vi "Main.vi"() -> ()   [LabVIEW 2018] (continued)
                    n1254 = call "SQL_Update.vi"("查询语句"=w6511, "表名"="Online", "error in (no error)"=w6514, "列名对应的值"=w6512, "列名"=string[] ["Last_Station", "Last_Result", "ST602_Date", "ST602_Time", "ST602_Result", "ST602_PanelNumber"], "connection reference"=w6513) -> ("error out"=w6510:errorcluster)  [unwired: 4 in, 1 out]
                    n1255 = Unbundle By Name(w6510) -> ("status"=w6518:bool)
                    n1256 = Equal?(x=w6509, y="") -> (x = y?=w6516:bool)
                    n1257 = Or(x=w6518, y=w6516) -> (x .or. y?=w6515:bool)
                    n1258 = case shown="假" w6515 {
                      tunnel: ["1" ("数据保存请求回复") "2" ("数据保存请求回复")] -> w6508
                      frame False {
                      }
                      frame True {
                      }
                    }
                  }
                  frame True {
                    n1259 = Delete From Array(array=w6539, length=2 ("长度"), index=0 ("索引")) -> (deleted portion=w6527:string[], array with subset deleted=w6536:string[])
                    n1260 = call "SQL_Update.vi"("查询语句"=w6524, "表名"="Online", "error in (no error)"=w6532, "列名对应的值"=w6527, "列名"=string[] ["Last_Station", "Last_Result"], "connection reference"=w6533) -> ("error out"=w6531:errorcluster, "connection reference 2"=w6530:T5)  [unwired: 4 in]
                    n1261 = call "SQL_Update.vi"("查询语句"=w6524, "表名"="Rework", "error in (no error)"=w6531, "列名对应的值"=w6536, "列名"=string[] ["ST602_Date", "ST602_Time", "ST602_Result", "ST602_PanelNumber"], "connection reference"=w6530) -> ("error out"=w6525:errorcluster)  [unwired: 4 in, 1 out]
                    n1262 = Unbundle By Name(w6525) -> ("status"=w6542:bool)
                    n1263 = Equal?(x="", y=w6534) -> (x = y?=w6541:bool)
                    n1264 = Or(x=w6542, y=w6541) -> (x .or. y?=w6540:bool)
                    n1265 = case shown="真" w6540 {
                      tunnel: ["1" ("数据保存请求回复") "2" ("数据保存请求回复")] -> w6526
                      frame False {
                      }
                      frame True {
                      }
                    }
                  }
                }
              }
            }
            "数据保存请求回复602" <- w6455
            n1266 = Delete From Array(array=w6443, length=2 ("长度"), index=0 ("索引")) -> (array with subset deleted=w6450:string[])  [unwired: 1 out]
            n1267 = local write "602数据回复输入"(w6454) -> ()
            n1268 = Insert Into Array(array=w6450, index=2 ("索引"), new element=w6442) -> (w6449:string[])
            n1269 = Insert Into Array(array=string[][] [] ("数组"), index (row)=0 ("索引 (行)"), new element=w6449) -> (w6451:string[][])  [unwired: 1 in]
            n1270 = Transpose 2D Array(2D array=w6451) -> (transposed array=w6441:string[][])
            n1271 = property on="ST602_DATA" class="MCListbox (严格)"("ItemNames"=w6441) -> ()  [unwired: 2 in, 2 out]
            "ST602数据读取（事件）" <- FALSE ("ST602数据读取（事件）")
          }
          event "ST603扫码请求（事件）": Value Change {
            n1272 = event-data() -> ()  [unwired: 1 in, 2 out]
            n1273 = local read "603二维码"() -> (w6548:string)
            n1274 = Concatenate Strings("Where QRCode='" ("查询语句"), w6548, "'" ("字符串")) -> (w6559:string)
            n1275 = call "SQL_Select.vi"("要读取的列名"=string[] ["Last_Station", "Last_Result"], "表名"="Online", "error in (no error)"=w6551, "查询语句"=w6559, "查询条件"=TRUE, "connection reference"=w6552) -> ("error out"=w6550:errorcluster, "数据"=w6558:string[][])  [unwired: 3 in, 1 out]
            n1276 = case shown="无错误" w6550 {
              tunnel: w6558 -> [w6568 _]
              tunnel: ["1" ("右扫码请求回复") "2" ("右扫码请求回复")] -> w6547
              tunnel: [TRUE TRUE] -> w6546
              frame No Error {
                n1277 = Index Array(array=w6568, index (row)=0 ("索引 (行)")) -> (element=w6565:string[])  [unwired: 1 in]
                n1278 = Index Array(array=w6565, index #1=0 ("索引 (行)")) -> (element #1=→"上一站号 (603)":string, element #2=→"上一站结果 (603)":string)  [unwired: 1 in]
              }
              frame Error {
              }
            }
            "扫码请求回复603" <- w6547
            n1279 = local write "603扫码回复输入"(w6546) -> ()
            "ST603扫码请求（事件）" <- FALSE ("ST603扫码请求（事件）")
          }
          event "ST603数据读取（事件）": Value Change {
            w6593 = 0 ("索引 (行)")
            n1280 = event-data() -> ()  [unwired: 1 in, 2 out]
            n1281 = local read "603二维码"() -> (w6572:string)
            n1282 = Concatenate Strings("Where QRCode='" ("查询语句"), w6572, "'" ("字符串")) -> (w6600:string)
            n1283 = call "SQL_Select.vi"("要读取的列名"=string[] ["Rework_Status"], "表名"="Online", "error in (no error)"=w6586, "查询语句"=w6600, "查询条件"=TRUE, "connection reference"=w6587) -> ("error out"=w6595:errorcluster, "数据"=w6599:string[][], "connection reference out"=w6596:T5)  [unwired: 3 in]
            n1284 = Index Array(array=w6599, index (row)=w6593, index (col)=w6593) -> (element=w6598:string)
            n1285 = Equal?(x=w6598, y="T") -> (x = y?=w6597:bool)
            n1286 = local read "603data"() -> (w6573:string[])
            n1287 = case shown="假" w6597 {
              tunnel: [w6614 w6620] -> w6585
              tunnel: w6573 -> [w6613 w6623]
              tunnel: [w6608 w6619] -> w6583
              tunnel: w6572 -> [w6607 w6622]
              tunnel: w6600 -> [w6606 w6621]
              tunnel: w6596 -> [w6605 w6634]
              tunnel: w6595 -> [w6604 w6633]
              tunnel: [TRUE w6618] -> w6584
              frame False {
                n1288 = call "SQL_Update.vi"("查询语句"=w6606, "表名"="Online", "error in (no error)"=w6604, "列名对应的值"=w6613, "列名"=string[] ["Last_Station", "Last_Result", "ST603_Date", "ST603_Time", "ST603_Result", "ST603_PanelNumber", "ST603_Spring_Retainer_5020834", "ST603_Spring_5024602", "ST603_Retaining_ring_5018568", "ST603_Disc_spring_5005082", "ST603_Bushing_5024673"], "connection reference"=w6605) -> ("error out"=w6608:errorcluster)  [unwired: 4 in, 1 out]
                n1289 = Unbundle By Name(w6608) -> ("status"=w6612:bool)
                n1290 = Equal?(x=w6607, y="") -> (x = y?=w6610:bool)
                n1291 = Or(x=w6612, y=w6610) -> (x .or. y?=w6609:bool)
                n1292 = case shown="假" w6609 {
                  tunnel: ["1" ("数据保存请求回复") "2" ("数据保存请求回复")] -> w6614
                  frame False {
                  }
                  frame True {
                  }
                }
              }
              frame True {
                w6629 = 0 ("索引 (行)")
                n1293 = call "SQL_Select.vi"("要读取的列名"=string[] ["[603]"], "表名"="Rework_List", "error in (no error)"=w6633, "查询语句"=w6621, "查询条件"=TRUE, "connection reference"=w6634) -> ("error out"=w6624:errorcluster, "数据"=w6630:string[][], "connection reference out"=w6625:T5)  [unwired: 3 in]
                n1294 = Index Array(array=w6630, index (row)=w6629, index (col)=w6629) -> (element=w6628:string)
                n1295 = Equal?(x=w6628, y="T") -> (x = y?=w6626:bool)
                n1296 = case shown="真" w6626 {
                  tunnel: w6625 -> [w6643 w6663]
                  tunnel: w6624 -> [w6644 w6662]
                  tunnel: w6623 -> [w6642 w6669]
                  tunnel: w6622 -> [w6639 w6664]
                  tunnel: w6621 -> [w6641 w6654]
                  tunnel: [w6638 w6656] -> w6620
                  tunnel: [w6640 w6655] -> w6619
                  tunnel: [TRUE TRUE] -> w6618
                  frame False {
                    n1297 = call "SQL_Update.vi"("查询语句"=w6641, "表名"="Online", "error in (no error)"=w6644, "列名对应的值"=w6642, "列名"=string[] ["Last_Station", "Last_Result", "ST603_Date", "ST603_Time", "ST603_Result", "ST603_PanelNumber", "ST603_Spring_Retainer_5020834", "ST603_Spring_5024602", "ST603_Retaining_ring_5018568", "ST603_Disc_spring_5005082", "ST603_Bushing_5024673"], "connection reference"=w6643) -> ("error out"=w6640:errorcluster)  [unwired: 4 in, 1 out]
                    n1298 = Unbundle By Name(w6640) -> ("status"=w6648:bool)
                    n1299 = Equal?(x=w6639, y="") -> (x = y?=w6646:bool)
                    n1300 = Or(x=w6648, y=w6646) -> (x .or. y?=w6645:bool)
                    n1301 = case shown="假" w6645 {
                      tunnel: ["1" ("数据保存请求回复") "2" ("数据保存请求回复")] -> w6638
                      frame False {
                      }
                      frame True {
                      }
                    }
                  }
                  frame True {
                    n1302 = Delete From Array(array=w6669, length=2 ("长度"), index=0 ("索引")) -> (deleted portion=w6657:string[], array with subset deleted=w6666:string[])
                    n1303 = call "SQL_Update.vi"("查询语句"=w6654, "表名"="Online", "error in (no error)"=w6662, "列名对应的值"=w6657, "列名"=string[] ["Last_Station", "Last_Result"], "connection reference"=w6663) -> ("error out"=w6661:errorcluster, "connection reference 2"=w6660:T5)  [unwired: 4 in]
                    n1304 = call "SQL_Update.vi"("查询语句"=w6654, "表名"="Rework", "error in (no error)"=w6661, "列名对应的值"=w6666, "列名"=string[] ["ST603_Date", "ST603_Time", "ST603_Result", "ST603_PanelNumber", "ST603_Spring_Retainer_5020834", "ST603_Spring_5024602", "ST603_Retaining_ring_5018568", "ST603_Disc_spring_5005082", "ST603_Bushing_5024673"], "connection reference"=w6660) -> ("error out"=w6655:errorcluster)  [unwired: 4 in, 1 out]
                    n1305 = Unbundle By Name(w6655) -> ("status"=w6672:bool)
                    n1306 = Equal?(x="", y=w6664) -> (x = y?=w6671:bool)
                    n1307 = Or(x=w6672, y=w6671) -> (x .or. y?=w6670:bool)
                    n1308 = case shown="真" w6670 {
                      tunnel: ["1" ("数据保存请求回复") "2" ("数据保存请求回复")] -> w6656
                      frame False {
                      }
                      frame True {
                      }
                    }
                  }
                }
              }
            }
            "数据保存请求回复603" <- w6585
            n1309 = local write "603数据回复输入"(w6584) -> ()
            n1310 = Delete From Array(array=w6573, length=2 ("长度"), index=0 ("索引")) -> (array with subset deleted=w6580:string[])  [unwired: 1 out]
            n1311 = Insert Into Array(array=w6580, index=2 ("索引"), new element=w6572) -> (w6579:string[])
            n1312 = Insert Into Array(array=string[][] [] ("数组"), index (row)=0 ("索引 (行)"), new element=w6579) -> (w6581:string[][])  [unwired: 1 in]
            n1313 = Transpose 2D Array(2D array=w6581) -> (transposed array=w6571:string[][])
            n1314 = property on="ST603_DATA" class="MCListbox (严格)"("ItemNames"=w6571) -> ()  [unwired: 2 in, 2 out]
            "ST603数据读取（事件）" <- FALSE ("ST603数据读取（事件）")
          }
          event "ST70数据读取（事件）", "ST70数据读取（事件） 2": Value Change {
            w6696 = 0 ("索引 (行)")
            w6703 = "ST70" ("表名")
            n1315 = event-data() -> ("CtlRef"=w6678:refnum<vi>)  [unwired: 1 in, 1 out]
            n1316 = property class="Bool (严格)"(reference=w6678) -> ("Label.Text"=w6677:string)  [unwired: 1 in, 2 out]
            n1317 = case shown="\"ST70数据读取（事件）\", 默认" w6677 {
              tunnel: ["70数据 2-手动测试" w6727] -> w6701
              frame "ST70数据读取（事件） 2" {
              }
              frame "ST70数据读取（事件）", Default {
                n1318 = local read "70数据"() -> (w6727:string[])
              }
            }
            n1319 = Format Date/Time String(time format string (%c)="%Y-%m-%d_%H-%M-%S" ("时间格式字符串(%c)")) -> (date/time string=w6681:string)  [unwired: 2 in]
            n1320 = call "SQL_Insert.vi"("表名"=w6703, "error in (no error)"=w6714, "值"=w6701, "列名"=string[] ["ST70_Number", "Last_Station", "Last_Result", "ST70_Date", "ST70_Time", "ST70_Result", "ST70_Pressure_Final1", "ST70_Distance_Final1", "ST70_Pressure_Upper1", "ST70_Pressure_Lower1", "ST70_Distance_Upper1", "ST70_Distance_Lower1", "ST70_Pressure_Final2", "ST70_Distance_Final2", "ST70_Pressure_Upper2", "ST70_Pressure_Lower2", "ST70_Distance_Upper2", "ST70_Distance_Lower2", "ST70_Inflexion_force_Left_Final", "ST70_Inflexion_force_Left_Upper", "ST70_Inflexion_force_Left_Lower", "ST70_Inflexion_force_Right_Final", "ST70_Inflexion_force_Right_Upper", "ST70_Inflexion_force_Right_Lower", "ST70_Housing_5025351", "ST70_Bushing_5025400"], "connection reference"=w6715) -> ("error out"=w6704:errorcluster, "connection reference 2"=w6702:T5)  [unwired: 5 in]
            n1321 = Index Array(array=w6701, index #1=0 ("索引"), index #2=3 ("索引"), index #3=4 ("索引")) -> (element #1=w6688:string, element #2=w6686:string, element #3=w6685:string)
            n1322 = Concatenate Strings("Where ST70_Number='" ("查询语句"), w6688, "'" ("字符串")) -> (w6699:string)
            n1323 = call "SQL_Select.vi"("表名"=w6703, "error in (no error)"=w6704, "查询语句"=w6699, "查询条件"=TRUE, "connection reference"=w6702) -> ("error out"=w6680:errorcluster, "数据"=w6697:string[][])  [unwired: 4 in, 1 out]
            n1324 = Unbundle By Name(w6680) -> ("source"=w6679:string)
            n1325 = Concatenate Strings(w6688, "----" ("字符串"), w6686, w6685, "———" ("字符串"), w6681, w6679) -> (w6684:string)
            n1326 = Unbundle By Name(w6680) -> ("status"=w6698:bool)
            n1327 = Index Array(array=w6697, index (row)=w6696, index (col)=w6696) -> (element=w6694:string)
            n1328 = disable-structure shown="禁用" {
              disable-tunnel: w6684 -> [w6716 _]
              frame Disabled {
                n1329 = disable-structure shown="启用" {
                  disable-tunnel: w6716 -> [w6719 w6721]
                  frame Disabled {
                    n1330 = local read "70数据"() -> (w6720:string[])
                    n1331 = Insert Into Array(array=w6720, new element=w6719) -> (w6718:string[])  [unwired: 1 in]
                    n1332 = local write "70数据"(w6718) -> ()
                    n1333 = Write to Text File(file (use dialog)=path "D:/70数据.txt" ("文件（使用对话框）"), text=w6718) -> ()  [unwired: 2 in, 3 out]
                  }
                  frame Enabled {
                    n1334 = call "站点编码更新（年月日）.vi"("当前编码信息"=w6721, "站别"="70") -> ()  [unwired: 10 in]
                  }
                }
              }
              frame Enabled {
              }
            }
            n1335 = call <vilib>:"Trim Whitespace.vi"("string"=w6694) -> ("trimmed string"=w6693:string)  [unwired: 1 in]
            n1336 = Equal?(x=w6693, y="") -> (x = y?=w6695:bool)
            n1337 = Insert Into Array(array=string[][] [] ("数组"), index (row)=0 ("索引 (行)"), new element=w6701) -> (w6710:string[][])  [unwired: 1 in]
            n1338 = Or(x=w6698, y=w6695) -> (x .or. y?=w6676:bool)
            n1339 = Transpose 2D Array(2D array=w6710) -> (transposed array=w6707:string[][])
            n1340 = property on="ST70_DATA" class="MCListbox (严格)"("ItemNames"=w6707) -> ()  [unwired: 2 in, 2 out]
            n1341 = case shown="真" w6676 {
              frame False {
                n1342 = property on="ST70画曲线" class="Bool (严格)"("Val(Sgnl)"=TRUE ("值(信号)")) -> ()  [unwired: 2 in, 2 out]
              }
              frame True {
                n1343 = local write "70数据回复输入"(TRUE) -> ()
                "数据保存请求回复70" <- "2" ("数据保存请求回复")
              }
            }
            "ST70数据读取（事件）" <- FALSE ("ST70数据读取（事件）")
          }
          event "ST80扫码请求 （事件）": Value Change {
            n1344 = event-data() -> ()  [unwired: 1 in, 2 out]
            n1345 = local read "80二维码"() -> (w6732:string)
            n1346 = Concatenate Strings("Where QRCode='" ("查询语句"), w6732, "'" ("字符串")) -> (w6741:string)
            n1347 = call "SQL_Select.vi"("要读取的列名"=string[] ["Last_Station", "Last_Result"], "表名"="Online", "error in (no error)"=w6733, "查询语句"=w6741, "查询条件"=TRUE, "connection reference"=w6734) -> ("error out"=w6731:errorcluster, "数据"=w6740:string[][])  [unwired: 3 in, 1 out]
            n1348 = case shown="无错误" w6731 {
              tunnel: w6740 -> [w6750 _]
              tunnel: ["1" ("右扫码请求回复") "2" ("右扫码请求回复")] -> w6730
              tunnel: [TRUE TRUE] -> w6729
              frame No Error {
                n1349 = Index Array(array=w6750, index (row)=0 ("索引 (行)")) -> (element=w6747:string[])  [unwired: 1 in]
                n1350 = Index Array(array=w6747, index #1=0 ("索引 (行)")) -> (element #1=→"上一站号 (80)":string, element #2=→"上一站结果 (80)":string)  [unwired: 1 in]
              }
              frame Error {
              }
            }
            "扫码请求回复80" <- w6730
            n1351 = local write "80扫码回复写入"(w6729) -> ()
            "ST80扫码请求 （事件）" <- FALSE ("ST80扫码请求 （事件）")
          }
          event "ST80数据保存请求（事件）": Value Change {
            w6775 = 0 ("索引 (行)")
            n1352 = event-data() -> ()  [unwired: 1 in, 2 out]
            n1353 = local read "80二维码"() -> (w6754:string)
            n1354 = Concatenate Strings("Where QRCode='" ("查询语句"), w6754, "'" ("字符串")) -> (w6782:string)
            n1355 = call "SQL_Select.vi"("要读取的列名"=string[] ["Rework_Status"], "表名"="Online", "error in (no error)"=w6768, "查询语句"=w6782, "查询条件"=TRUE, "connection reference"=w6769) -> ("error out"=w6777:errorcluster, "数据"=w6781:string[][], "connection reference out"=w6778:T5)  [unwired: 3 in]
            n1356 = Index Array(array=w6781, index (row)=w6775, index (col)=w6775) -> (element=w6780:string)
            n1357 = Equal?(x=w6780, y="T") -> (x = y?=w6779:bool)
            n1358 = local read "80数据"() -> (w6755:string[])
            n1359 = case shown="真" w6779 {
              tunnel: [w6796 w6802] -> w6767
              tunnel: w6755 -> [w6795 w6805]
              tunnel: [w6790 w6801] -> w6765
              tunnel: w6754 -> [w6789 w6804]
              tunnel: w6782 -> [w6788 w6803]
              tunnel: w6778 -> [w6787 w6816]
              tunnel: w6777 -> [w6786 w6815]
              tunnel: [TRUE w6800] -> w6766
              frame False {
                n1360 = call "SQL_Update.vi"("查询语句"=w6788, "表名"="Online", "error in (no error)"=w6786, "列名对应的值"=w6795, "列名"=string[] ["Last_Station", "Last_Result", "ST80_Date", "ST80_Time", "ST80_Result", "ST80_Flat_Sael_5020064", "ST80_Spring_5024883", "ST80_Spring_Plate_5025473"], "connection reference"=w6787) -> ("error out"=w6790:errorcluster)  [unwired: 4 in, 1 out]
                n1361 = Unbundle By Name(w6790) -> ("status"=w6794:bool)
                n1362 = Equal?(x=w6789, y="") -> (x = y?=w6792:bool)
                n1363 = Or(x=w6794, y=w6792) -> (x .or. y?=w6791:bool)
                n1364 = case shown="假" w6791 {
                  tunnel: ["1" ("数据保存请求回复") "2" ("数据保存请求回复")] -> w6796
                  frame False {
                  }
                  frame True {
                  }
                }
              }
              frame True {
                w6811 = 0 ("索引 (行)")
                n1365 = call "SQL_Select.vi"("要读取的列名"=string[] ["[80]"], "表名"="Rework_List", "error in (no error)"=w6815, "查询语句"=w6803, "查询条件"=TRUE, "connection reference"=w6816) -> ("error out"=w6806:errorcluster, "数据"=w6812:string[][], "connection reference out"=w6807:T5)  [unwired: 3 in]
                n1366 = Index Array(array=w6812, index (row)=w6811, index (col)=w6811) -> (element=w6810:string)
                n1367 = Equal?(x=w6810, y="T") -> (x = y?=w6808:bool)
                n1368 = case shown="真" w6808 {
                  tunnel: w6807 -> [w6825 w6845]
                  tunnel: w6806 -> [w6826 w6844]
                  tunnel: w6805 -> [w6824 w6851]
                  tunnel: w6804 -> [w6821 w6846]
                  tunnel: w6803 -> [w6823 w6836]
                  tunnel: [w6820 w6838] -> w6802
                  tunnel: [w6822 w6837] -> w6801
                  tunnel: [TRUE TRUE] -> w6800
                  frame False {
                    n1369 = call "SQL_Update.vi"("查询语句"=w6823, "表名"="Online", "error in (no error)"=w6826, "列名对应的值"=w6824, "列名"=string[] ["Last_Station", "Last_Result", "ST80_Date", "ST80_Time", "ST80_Result", "ST80_Flat_Sael_5020064", "ST80_Spring_5024883", "ST80_Spring_Plate_5025473"], "connection reference"=w6825) -> ("error out"=w6822:errorcluster)  [unwired: 4 in, 1 out]
                    n1370 = Unbundle By Name(w6822) -> ("status"=w6830:bool)
                    n1371 = Equal?(x=w6821, y="") -> (x = y?=w6828:bool)
                    n1372 = Or(x=w6830, y=w6828) -> (x .or. y?=w6827:bool)
                    n1373 = case shown="假" w6827 {
                      tunnel: ["1" ("数据保存请求回复") "2" ("数据保存请求回复")] -> w6820
                      frame False {
                      }
                      frame True {
                      }
                    }
                  }
                  frame True {
                    n1374 = Delete From Array(array=w6851, length=2 ("长度"), index=0 ("索引")) -> (deleted portion=w6839:string[], array with subset deleted=w6848:string[])
                    n1375 = call "SQL_Update.vi"("查询语句"=w6836, "表名"="Online", "error in (no error)"=w6844, "列名对应的值"=w6839, "列名"=string[] ["Last_Station", "Last_Result"], "connection reference"=w6845) -> ("error out"=w6843:errorcluster, "connection reference 2"=w6842:T5)  [unwired: 4 in]
                    n1376 = call "SQL_Update.vi"("查询语句"=w6836, "表名"="Rework", "error in (no error)"=w6843, "列名对应的值"=w6848, "列名"=string[] ["ST80_Date", "ST80_Time", "ST80_Result", "ST80_Flat_Sael_5020064", "ST80_Spring_5024883", "ST80_Spring_Plate_5025473"], "connection reference"=w6842) -> ("error out"=w6837:errorcluster)  [unwired: 4 in, 1 out]
                    n1377 = Unbundle By Name(w6837) -> ("status"=w6854:bool)
                    n1378 = Equal?(x="", y=w6846) -> (x = y?=w6853:bool)
                    n1379 = Or(x=w6854, y=w6853) -> (x .or. y?=w6852:bool)
                    n1380 = case shown="真" w6852 {
                      tunnel: ["1" ("数据保存请求回复") "2" ("数据保存请求回复")] -> w6838
                      frame False {
                      }
                      frame True {
                      }
                    }
                  }
                }
              }
            }
            "数据保存请求回复80" <- w6767
            n1381 = Delete From Array(array=w6755, length=2 ("长度"), index=0 ("索引")) -> (array with subset deleted=w6762:string[])  [unwired: 1 out]
            n1382 = Insert Into Array(array=w6762, index=2 ("索引"), new element=w6754) -> (w6761:string[])
            n1383 = Insert Into Array(array=string[][] [] ("数组"), index (row)=0 ("索引 (行)"), new element=w6761) -> (w6763:string[][])  [unwired: 1 in]
            n1384 = Transpose 2D Array(2D array=w6763) -> (transposed array=w6753:string[][])
            n1385 = property on="ST80_DATA" class="MCListbox (严格)"("ItemNames"=w6753) -> ()  [unwired: 2 in, 2 out]
            n1386 = local write "80数据回复写入"(w6766) -> ()
            "ST80数据保存请求（事件）" <- FALSE ("ST80数据保存请求（事件）")
          }
          event "ST901扫码请求（事件）": Value Change {
            w6859 = path "D:/BOSCH/OP90/CH_00_1/PRG_00" ("路径")
            n1387 = event-data() -> ()  [unwired: 1 in, 2 out]
            n1388 = List Folder(path=w6859) -> (filenames=w6858:string[])  [unwired: 3 in, 3 out]
            n1389 = for {
              tunnel: w6858 -> [w6877] mode=indexing
              tunnel: w6859 -> [w6878]
              n1390 = Build Path(base path=w6878, name or relative path=w6877) -> (appended path=w6875:path)
              n1391 = Delete(path (use dialog)=w6875, entire hierarchy (F)=TRUE ("整个层次结构(F)")) -> ()  [unwired: 3 in, 3 out]
            }
            n1392 = local read "901二维码"() -> (w6862:string)
            n1393 = Concatenate Strings("Where QRCode='" ("查询语句"), w6862, "'" ("字符串")) -> (w6873:string)
            n1394 = call "SQL_Select.vi"("要读取的列名"=string[] ["Last_Station", "Last_Result"], "表名"="Online", "error in (no error)"=w6865, "查询语句"=w6873, "查询条件"=TRUE, "connection reference"=w6866) -> ("error out"=w6864:errorcluster, "数据"=w6872:string[][])  [unwired: 3 in, 1 out]
            n1395 = case shown="无错误" w6864 {
              tunnel: w6872 -> [w6886 _]
              tunnel: ["1" ("右扫码请求回复") "2" ("右扫码请求回复")] -> w6861
              tunnel: [TRUE TRUE] -> w6860
              frame No Error {
                n1396 = Index Array(array=w6886, index (row)=0 ("索引 (行)")) -> (element=w6883:string[])  [unwired: 1 in]
                n1397 = Index Array(array=w6883, index #1=0 ("索引 (行)")) -> (element #1=→"上一站号 (901)":string, element #2=→"上一站结果 (901)":string)  [unwired: 1 in]
              }
              frame Error {
              }
            }
            "扫码请求回复901" <- w6861
            n1398 = local write "901扫码回复输入"(w6860) -> ()
            "ST901扫码请求（事件）" <- FALSE ("ST901扫码请求（事件）")
          }
          event "ST901数据读取（事件）": Value Change {
            # "扫码-扫码请求--80站状态---编码--编码请求--70站判断----读取"
            n1399 = event-data() -> ()  [unwired: 1 in, 2 out]
            n1400 = local read "901编码"() -> (w6899:string)
            n1401 = Concatenate Strings("Where ST70_Number='" ("查询语句"), w6899, "'" ("字符串")) -> (w6897:string)
            n1402 = call "SQL_Select.vi"("要读取的列名"=string[] ["ST70_Number", "ST70_Date", "ST70_Time", "ST70_Result", "ST70_Pressure_Final1", "ST70_Pressure_Upper1", "ST70_Pressure_Lower1", "ST70_Distance_Final1", "ST70_Distance_Upper1", "ST70_Distance_Lower1", "ST70_Pressure_Final2", "ST70_Pressure_Upper2", "ST70_Pressure_Lower2", "ST70_Distance_Final2", "ST70_Distance_Upper2", "ST70_Distance_Lower2", "ST70_Inflexion_force_Left_Final", "ST70_Inflexion_force_Left_Upper", "ST70_Inflexion_force_Left_Lower", "ST70_Inflexion_force_Right_Final", "ST70_Inflexion_force_Right_Upper", "ST70_Inflexion_force_Right_Lower", "ST70_Housing_5025351", "ST70_Bushing_5025400"], "表名"="ST70", "查询语句"=w6897, "查询条件"=TRUE, "connection reference"=w6901) -> ("error out"=w6894:errorcluster, "数据"=w6893:string[][], "connection reference out"=w6895:T5)  [unwired: 4 in]
            n1403 = local read "901二维码"() -> (w6890:string)
            n1404 = Not Equal?(x=w6890, y="") -> (x != y?=w6889:bool)
            n1405 = Concatenate Strings("Where QRCode='" ("查询语句"), w6890, "'" ("字符串")) -> (w6908:string)
            n1406 = case shown="真" w6889 {
              tunnel: w6908 -> [_ w6918]
              tunnel: [errorcluster {"status"=TRUE, "code"=0, "source"="，二维码为空"} ("error out") w6912] -> w6905
              tunnel: w6895 -> [_ w6940]
              tunnel: w6894 -> [_ w6939]
              tunnel: w6893 -> [_ w6937]
              tunnel: [TRUE w6915] -> w6892
              tunnel: w6890 -> [_ w6925]
              frame False {
              }
              frame True {
                w6944 = 0 ("索引 (行)")
                n1407 = call "SQL_Select.vi"("要读取的列名"=string[] ["Rework_Status"], "表名"="Online", "error in (no error)"=w6939, "查询语句"=w6918, "查询条件"=TRUE, "connection reference"=w6940) -> ("error out"=w6919:errorcluster, "数据"=w6947:string[][], "connection reference out"=w6920:T5)  [unwired: 3 in]
                n1408 = local read "901数据"() -> (w6916:string[])
                n1409 = Index Array(array=w6947, index (row)=w6944, index (col)=w6944) -> (element=w6946:string)
                n1410 = Equal?(x=w6946, y="T") -> (x = y?=w6921:bool)
                n1411 = flat-sequence {
                  tunnel: w6918 -> [w6957]
                  tunnel: w6920 -> [w6956]
                  tunnel: w6919 -> [w6955]
                  tunnel: w6917 -> [w6953]
                  tunnel: [w6954] -> w6924
                  tunnel: [w6952] -> w6923
                  tunnel: [w6951] -> w6922
                  tunnel: w6921 -> [w6950]
                  tunnel: [w6949] -> w6914
                  tunnel: [w6948] -> w6913
                  tunnel: w6924 -> [w7016]
                  tunnel: w6923 -> [w7011]
                  tunnel: w6922 -> [w7017]
                  tunnel: [w7015] -> w6915
                  tunnel: w6914 -> [w7014]
                  tunnel: w6913 -> [w7010]
                  tunnel: [w7009] -> w6912
                  frame #0 {
                    n1412 = case shown="真" w6950 {
                      tunnel: w6953 -> [w6958 w6973]
                      tunnel: [w6965 w6971] -> w6954
                      tunnel: w6957 -> [w6960 w6972]
                      tunnel: w6956 -> [w6964 w6983]
                      tunnel: w6955 -> [w6963 w6982]
                      tunnel: [w6961 w6970] -> w6951
                      tunnel: [w6960 w6969] -> w6952
                      tunnel: [FALSE w6968] -> w6949
                      tunnel: [w6958 w6967] -> w6948
                      frame False {
                        n1413 = call "SQL_Update.vi"("查询语句"=w6960, "表名"="Online", "error in (no error)"=w6963, "列名对应的值"=w6958, "列名"=string[] ["Last_Station", "Last_Result", "ST901_Date", "ST901_Time", "ST901_Result", "ST901_Torque1", "ST901_Angle1", "ST901_Torque2", "ST901_Angle2", "ST901_Torque3", "ST901_Angle3", "ST901_Torque4", "ST901_Angle4", "ST901_Torque5", "ST901_Angle5", "ST901_Torque_Upper", "ST901_Torque_Lower", "ST901_Angle_Upper", "ST901_Angle_Lower", "ST901_Gradient1", "ST901_Gradient2", "ST901_Gradient3", "ST901_Gradient4", "ST901_Gradient5", "ST901_Gradient_Upper", "ST901_Gradient_Lower", "ST70_Number", "ST70_Date", "ST70_Time", "ST70_Result", "ST70_Pressure_Final1", "ST70_Pressure_Upper1", "ST70_Pressure_Lower1", "ST70_Distance_Final1", "ST70_Distance_Upper1", "ST70_Distance_Lower1", "ST70_Pressure_Final2", "ST70_Pressure_Upper2", "ST70_Pressure_Lower2", "ST70_Distance_Final2", "ST70_Distance_Upper2", "ST70_Distance_Lower2", "ST70_Inflexion_force_Left_Final", "ST70_Inflexion_force_Left_Upper", "ST70_Inflexion_force_Left_Lower", "ST70_Inflexion_force_Right_Final", "ST70_Inflexion_force_Right_Upper", "ST70_Inflexion_force_Right_Lower", "ST70_Housing_5025351", "ST70_Bushing_5025400"] ("输出数组"), "connection reference"=w6964) -> ("error out"=w6965:errorcluster, "connection reference 2"=w6961:T5)  [unwired: 4 in]
                      }
                      frame True {
                        w6978 = 0 ("索引 (行)")
                        n1414 = call "SQL_Select.vi"("要读取的列名"=string[] ["[901]"], "表名"="Rework_List", "error in (no error)"=w6982, "查询语句"=w6972, "查询条件"=TRUE, "connection reference"=w6983) -> ("error out"=w6974:errorcluster, "数据"=w6979:string[][], "connection reference out"=w6975:T5)  [unwired: 3 in]
                        n1415 = Index Array(array=w6979, index (row)=w6978, index (col)=w6978) -> (element=w6977:string)
                        n1416 = Equal?(x=w6977, y="T") -> (x = y?=w6968:bool)
                        n1417 = case shown="真" w6968 {
                          tunnel: w6975 -> [w6990 w7004]
                          tunnel: w6974 -> [w6991 w7003]
                          tunnel: w6973 -> [w6985 w7007]
                          tunnel: w6972 -> [w6987 w6994]
                          tunnel: [w6989 w6997] -> w6971
                          tunnel: [w6986 w6995] -> w6970
                          tunnel: [w6987 w6994] -> w6969
                          tunnel: [w6985 w6993] -> w6967
                          frame False {
                            n1418 = call "SQL_Update.vi"("查询语句"=w6987, "表名"="Online", "error in (no error)"=w6991, "列名对应的值"=w6985, "列名"=string[] ["Last_Station", "Last_Result", "ST901_Date", "ST901_Time", "ST901_Result", "ST901_Torque1", "ST901_Angle1", "ST901_Torque2", "ST901_Angle2", "ST901_Torque3", "ST901_Angle3", "ST901_Torque4", "ST901_Angle4", "ST901_Torque5", "ST901_Angle5", "ST901_Torque_Upper", "ST901_Torque_Lower", "ST901_Angle_Upper", "ST901_Angle_Lower", "ST901_Gradient1", "ST901_Gradient2", "ST901_Gradient3", "ST901_Gradient4", "ST901_Gradient5", "ST901_Gradient_Upper", "ST901_Gradient_Lower", "ST70_Number", "ST70_Date", "ST70_Time", "ST70_Result", "ST70_Pressure_Final1", "ST70_Pressure_Upper1", "ST70_Pressure_Lower1", "ST70_Distance_Final1", "ST70_Distance_Upper1", "ST70_Distance_Lower1", "ST70_Pressure_Final2", "ST70_Pressure_Upper2", "ST70_Pressure_Lower2", "ST70_Distance_Final2", "ST70_Distance_Upper2", "ST70_Distance_Lower2", "ST70_Inflexion_force_Left_Final", "ST70_Inflexion_force_Left_Upper", "ST70_Inflexion_force_Left_Lower", "ST70_Inflexion_force_Right_Final", "ST70_Inflexion_force_Right_Upper", "ST70_Inflexion_force_Right_Lower", "ST70_Housing_5025351", "ST70_Bushing_5025400"] ("输出数组"), "connection reference"=w6990) -> ("error out"=w6989:errorcluster, "connection reference 2"=w6986:T5)  [unwired: 4 in]
                          }
                          frame True {
                            n1419 = Delete From Array(array=w7007, length=2 ("长度"), index=0 ("索引")) -> (deleted portion=w6998:string[], array with subset deleted=w6993:string[])
                            n1420 = call "SQL_Update.vi"("查询语句"=w6994, "表名"="Online", "error in (no error)"=w7003, "列名对应的值"=w6998, "列名"=string[] ["Last_Station", "Last_Result"], "connection reference"=w7004) -> ("error out"=w7002:errorcluster, "connection reference 2"=w7001:T5)  [unwired: 4 in]
                            n1421 = call "SQL_Update.vi"("查询语句"=w6994, "表名"="Rework", "error in (no error)"=w7002, "列名对应的值"=w6993, "列名"=string[] ["ST901_Date", "ST901_Time", "ST901_Result", "ST901_Torque1", "ST901_Angle1", "ST901_Torque2", "ST901_Angle2", "ST901_Torque3", "ST901_Angle3", "ST901_Torque4", "ST901_Angle4", "ST901_Torque5", "ST901_Angle5", "ST901_Torque_Upper", "ST901_Torque_Lower", "ST901_Angle_Upper", "ST901_Angle_Lower", "ST901_Gradient1", "ST901_Gradient2", "ST901_Gradient3", "ST901_Gradient4", "ST901_Gradient5", "ST901_Gradient_Upper", "ST901_Gradient_Lower", "ST70_Number", "ST70_Date", "ST70_Time", "ST70_Result", "ST70_Pressure_Final1", "ST70_Pressure_Upper1", "ST70_Pressure_Lower1", "ST70_Distance_Final1", "ST70_Distance_Upper1", "ST70_Distance_Lower1", "ST70_Pressure_Final2", "ST70_Pressure_Upper2", "ST70_Pressure_Lower2", "ST70_Distance_Final2", "ST70_Distance_Upper2", "ST70_Distance_Lower2", "ST70_Inflexion_force_Left_Final", "ST70_Inflexion_force_Left_Upper", "ST70_Inflexion_force_Left_Lower", "ST70_Inflexion_force_Right_Final", "ST70_Inflexion_force_Right_Upper", "ST70_Inflexion_force_Right_Lower", "ST70_Housing_5025351", "ST70_Bushing_5025400"] ("输出数组"), "connection reference"=w7001) -> ("error out"=w6997:errorcluster, "connection reference 2"=w6995:T5)  [unwired: 4 in]
                          }
                        }
                      }
                    }
                  }
                  frame #1 {
                    w7021 = 0 ("索引 (行)")
                    n1422 = call "SQL_Select.vi"("要读取的列名"=string[] ["Last_Station"], "表名"="Online", "error in (no error)"=w7016, "查询语句"=w7011, "查询条件"=TRUE, "connection reference"=w7017) -> ("error out"=w7012:errorcluster, "数据"=w7022:string[][], "connection reference out"=w7013:T5)  [unwired: 3 in]
                    n1423 = Index Array(array=w7022, index (row)=w7021) -> (element=w7023:string[])  [unwired: 1 in]
                    n1424 = Index Array(array=w7023, index=w7021) -> (element=w7020:string)
                    n1425 = Equal?(x=w7020, y="901") -> (x = y?=w7018:bool)
                    n1426 = case shown="假" w7018 {
                      tunnel: [w7028 FALSE] -> w7015
                      tunnel: w7014 -> [w7044 _]
                      tunnel: w7013 -> [w7043 _]
                      tunnel: w7012 -> [w7042 _]
                      tunnel: w7011 -> [w7041 _]
                      tunnel: w7010 -> [w7040 _]
                      tunnel: [w7029 errorcluster {"status"=FALSE, "code"=0, "source"=""} ("error out")] -> w7009
                      frame False {
                        w7034 = 0 ("索引 (行)")
                        n1427 = case shown="真" w7044 {
                          tunnel: w7043 -> [w7050 w7063]
                          tunnel: w7042 -> [w7051 w7062]
                          tunnel: w7040 -> [w7049 w7067]
                          tunnel: w7041 -> [w7046 w7053]
                          tunnel: [w7048 w7056] -> w7031
                          tunnel: [w7045 w7054] -> w7030
                          tunnel: [w7046 w7053] -> w7027
                          frame False {
                            n1428 = call "SQL_Update.vi"("查询语句"=w7046, "表名"="Online", "error in (no error)"=w7051, "列名对应的值"=w7049, "列名"=string[] ["Last_Station", "Last_Result", "ST901_Date", "ST901_Time", "ST901_Result", "ST901_Torque1", "ST901_Angle1", "ST901_Torque2", "ST901_Angle2", "ST901_Torque3", "ST901_Angle3", "ST901_Torque4", "ST901_Angle4", "ST901_Torque5", "ST901_Angle5", "ST901_Torque_Upper", "ST901_Torque_Lower", "ST901_Angle_Upper", "ST901_Angle_Lower", "ST901_Gradient1", "ST901_Gradient2", "ST901_Gradient3", "ST901_Gradient4", "ST901_Gradient5", "ST901_Gradient_Upper", "ST901_Gradient_Lower", "ST70_Number", "ST70_Date", "ST70_Time", "ST70_Result", "ST70_Pressure_Final1", "ST70_Pressure_Upper1", "ST70_Pressure_Lower1", "ST70_Distance_Final1", "ST70_Distance_Upper1", "ST70_Distance_Lower1", "ST70_Pressure_Final2", "ST70_Pressure_Upper2", "ST70_Pressure_Lower2", "ST70_Distance_Final2", "ST70_Distance_Upper2", "ST70_Distance_Lower2", "ST70_Inflexion_force_Left_Final", "ST70_Inflexion_force_Left_Upper", "ST70_Inflexion_force_Left_Lower", "ST70_Inflexion_force_Right_Final", "ST70_Inflexion_force_Right_Upper", "ST70_Inflexion_force_Right_Lower", "ST70_Housing_5025351", "ST70_Bushing_5025400"] ("输出数组"), "connection reference"=w7050) -> ("error out"=w7048:errorcluster, "connection reference 2"=w7045:T5)  [unwired: 4 in]
                          }
                          frame True {
                            n1429 = Delete From Array(array=w7067, length=2 ("长度"), index=0 ("索引")) -> (deleted portion=w7057:string[], array with subset deleted=w7064:string[])
                            n1430 = call "SQL_Update.vi"("查询语句"=w7053, "表名"="Online", "error in (no error)"=w7062, "列名对应的值"=w7057, "列名"=string[] ["Last_Station", "Last_Result"], "connection reference"=w7063) -> ("error out"=w7061:errorcluster, "connection reference 2"=w7060:T5)  [unwired: 4 in]
                            n1431 = call "SQL_Update.vi"("查询语句"=w7053, "表名"="Rework", "error in (no error)"=w7061, "列名对应的值"=w7064, "列名"=string[] ["ST901_Date", "ST901_Time", "ST901_Result", "ST901_Torque1", "ST901_Angle1", "ST901_Torque2", "ST901_Angle2", "ST901_Torque3", "ST901_Angle3", "ST901_Torque4", "ST901_Angle4", "ST901_Torque5", "ST901_Angle5", "ST901_Torque_Upper", "ST901_Torque_Lower", "ST901_Angle_Upper", "ST901_Angle_Lower", "ST901_Gradient1", "ST901_Gradient2", "ST901_Gradient3", "ST901_Gradient4", "ST901_Gradient5", "ST901_Gradient_Upper", "ST901_Gradient_Lower", "ST70_Number", "ST70_Date", "ST70_Time", "ST70_Result", "ST70_Pressure_Final1", "ST70_Pressure_Upper1", "ST70_Pressure_Lower1", "ST70_Distance_Final1", "ST70_Distance_Upper1", "ST70_Distance_Lower1", "ST70_Pressure_Final2", "ST70_Pressure_Upper2", "ST70_Pressure_Lower2", "ST70_Distance_Final2", "ST70_Distance_Upper2", "ST70_Distance_Lower2", "ST70_Inflexion_force_Left_Final", "ST70_Inflexion_force_Left_Upper", "ST70_Inflexion_force_Left_Lower", "ST70_Inflexion_force_Right_Final", "ST70_Inflexion_force_Right_Upper", "ST70_Inflexion_force_Right_Lower", "ST70_Housing_5025351", "ST70_Bushing_5025400"] ("输出数组"), "connection reference"=w7060) -> ("error out"=w7056:errorcluster, "connection reference 2"=w7054:T5)  [unwired: 4 in]
                          }
                        }
                        n1432 = call "SQL_Select.vi"("要读取的列名"=string[] ["Last_Station"], "表名"="Online", "error in (no error)"=w7031, "查询语句"=w7027, "查询条件"=TRUE, "connection reference"=w7030) -> ("error out"=w7029:errorcluster, "数据"=w7035:string[][])  [unwired: 3 in, 1 out]
                        n1433 = Index Array(array=w7035, index (row)=w7034) -> (element=w7036:string[])  [unwired: 1 in]
                        n1434 = Index Array(array=w7036, index=w7034) -> (element=w7033:string)
                        n1435 = Not Equal?(x=w7033, y="901") -> (x != y?=w7028:bool)
                      }
                      frame True {
                      }
                    }
                  }
                }
                n1436 = Index Array(array=w6937, index (row)=0 ("索引 (行)")) -> (element=w6936:string[])  [unwired: 1 in]
                n1437 = Array Size(array=w6916) -> (size(s)=w6938:i32)
                n1438 = Insert Into Array(array=w6916, index=w6938, new element=w6936) -> (w6917:string[])
                n1439 = Delete From Array(array=w6916, length=2 ("长度"), index=0 ("索引")) -> (array with subset deleted=w6933:string[])  [unwired: 1 out]
                n1440 = Insert Into Array(array=w6933, index=2 ("索引"), new element=w6925) -> (w6932:string[])
                n1441 = Insert Into Array(array=string[][] [] ("数组"), index (row)=0 ("索引 (行)"), new element=w6932) -> (w6934:string[][])  [unwired: 1 in]
                n1442 = Transpose 2D Array(2D array=w6934) -> (transposed array=w6926:string[][])
                n1443 = property on="ST901_DATA" class="MCListbox (严格)"("ItemNames"=w6926) -> ()  [unwired: 2 in, 2 out]
              }
            }
            n1444 = case shown="假" w6892 {
              frame False {
                n1445 = property on="ST90画曲线" class="Bool (严格)"("Val(Sgnl)"=TRUE ("值(信号)")) -> ()  [unwired: 2 in, 2 out]
              }
              frame True {
                n1446 = flat-sequence {
                  frame #0 {
                    "数据保存请求回复901" <- "2" ("数据保存请求回复901")
                  }
                  frame #1 {
                    n1447 = local write "901数据回复输入"(TRUE ("901数据回复输入")) -> ()
                  }
                }
              }
            }
            "ST901数据读取（事件）" <- FALSE ("ST901数据读取（事件）")
          }
          event "ST901编码请求 （事件）": Value Change {
            w7076 = "----" ("字符串")
            n1448 = event-data() -> ()  [unwired: 1 in, 2 out]
            n1449 = local read "901编码"() -> (w7078:string)
            n1450 = Concatenate Strings("Where ST70_Number='" ("查询语句"), w7078, "'" ("字符串")) -> (w7092:string)
            n1451 = Format Date/Time String(time format string (%c)="%y-%m-%d_%H:%M:%S" ("时间格式字符串(%c)")) -> (date/time string=w7079:string)  [unwired: 2 in]
            n1452 = call "SQL_Select.vi"("要读取的列名"=string[] ["Last_Station", "Last_Result"], "表名"="ST70", "error in (no error)"=w7084, "查询语句"=w7092, "查询条件"=TRUE, "connection reference"=w7085) -> ("error out"=w7075:errorcluster, "数据"=w7091:string[][])  [unwired: 3 in, 1 out]
            n1453 = Unbundle By Name(w7075) -> ("source"=w7074:string)
            n1454 = Concatenate Strings(w7078, w7076, w7079, w7076, w7074) -> (w7077:string)
            n1455 = case shown="无错误" w7075 {
              tunnel: w7091 -> [w7103 _]
              tunnel: ["1" ("右扫码请求回复") "2" ("右扫码请求回复")] -> w7082
              tunnel: [TRUE TRUE] -> w7081
              frame No Error {
                n1456 = Index Array(array=w7103, index (row)=0 ("索引 (行)")) -> (element=w7100:string[])  [unwired: 1 in]
                n1457 = Index Array(array=w7100, index #1=0 ("索引 (行)")) -> (element #1=→"上一站号 (901) 编码":string, element #2=→"上一站结果 (901)编码":string)  [unwired: 1 in]
              }
              frame Error {
              }
            }
            "编码请求回复901" <- w7082
            n1458 = disable-structure shown="禁用" {
              disable-tunnel: w7077 -> [w7095 _]
              frame Disabled {
                n1459 = call "站点编码更新（年月日）.vi"("当前编码信息"=w7095, "站别"="90") -> ()  [unwired: 10 in]
              }
              frame Enabled {
              }
            }
            n1460 = local write "901编码回复输入"(w7081) -> ()
            "ST901编码请求 （事件）" <- FALSE ("ST901编码请求 （事件）")
          }
          event "ST902扫码请求（事件）": Value Change {
            w7107 = 0 ("索引 (行)")
            n1461 = event-data() -> ()  [unwired: 1 in, 2 out]
            n1462 = local read "902二维码"() -> (w7117:string)
            n1463 = Concatenate Strings("Where QRCode='" ("查询语句"), w7117, "'" ("字符串")) -> (w7111:string)
            n1464 = call "SQL_Select.vi"("要读取的列名"=string[] ["ST902"], "表名"="Time", "error in (no error)"=w7115, "查询语句"=w7111, "查询条件"=TRUE, "connection reference"=w7116) -> ("error out"=w7109:errorcluster, "数据"=w7108:string[][], "connection reference out"=w7110:T5)  [unwired: 3 in]
            n1465 = Index Array(array=w7108, index (row)=w7107, index (col)=w7107) -> (element=w7106:string)
            n1466 = call "SQL_Select.vi"("要读取的列名"=string[] ["Last_Station", "Last_Result"], "表名"="Online", "error in (no error)"=w7109, "查询语句"=w7111, "查询条件"=TRUE, "connection reference"=w7110) -> ("error out"=w7123:errorcluster, "数据"=w7127:string[][])  [unwired: 3 in, 1 out]
            n1467 = case shown="无错误" w7123 {
              tunnel: w7127 -> [w7137 _]
              tunnel: [w7129 "2" ("右扫码请求回复")] -> w7121
              tunnel: [TRUE TRUE] -> w7120
              tunnel: w7106 -> [w7130 _]
              frame No Error {
                n1468 = Index Array(array=w7137, index (row)=0 ("索引 (行)")) -> (element=w7134:string[])  [unwired: 1 in]
                n1469 = Index Array(array=w7134, index #1=0 ("索引 (行)")) -> (element #1=→"上一站号 (902)":string, element #2=→"上一站结果 (902)":string)  [unwired: 1 in]
                n1470 = case shown="\"假\", 默认" w7130 {
                  tunnel: ["1" ("右扫码请求回复") "3" ("右扫码请求回复")] -> w7129
                  frame "假", Default {
                  }
                  frame "3" {
                  }
                }
              }
              frame Error {
              }
            }
            "扫码请求回复902" <- w7121
            n1471 = local write "902扫码回复输入"(w7120) -> ()
            "ST902扫码请求（事件）" <- FALSE ("ST902扫码请求（事件）")
          }
          event "ST902数据读取（事件）": Value Change {
            w7148 = 0 ("索引 (行)")
            w7151 = "Time" ("表名")
            w7179 = 0 ("索引 (行)")
            n1472 = event-data() -> ()  [unwired: 1 in, 2 out]
            n1473 = local read "902二维码"() -> (w7150:string)
            n1474 = Concatenate Strings("Where QRCode='" ("查询语句"), w7150, "'" ("字符串")) -> (w7147:string)
            n1475 = call "SQL_Select.vi"("要读取的列名"=string[] ["ST902"], "表名"=w7151, "error in (no error)"=w7145, "查询语句"=w7147, "查询条件"=TRUE, "connection reference"=w7146) -> ("error out"=w7152:errorcluster, "数据"=w7149:string[][], "connection reference out"=w7153:T5)  [unwired: 3 in]
            n1476 = Index Array(array=w7149, index (row)=w7148, index (col)=w7148) -> (element=w7142:string)
            n1477 = Matrix Size(0:w7149) -> (1:w7154:i32)  [unwired: 1 out]
            n1478 = case shown="0" w7154 {
              tunnel: w7153 -> [w7197 w7211]
              tunnel: w7152 -> [w7196 w7210]
              tunnel: w7151 -> [w7195 w7209]
              tunnel: w7150 -> [w7192 _]
              tunnel: [w7189 w7199] -> w7144
              tunnel: [w7188 w7198] -> w7143
              tunnel: w7142 -> [_ w7207]
              tunnel: w7147 -> [_ w7200]
              frame 0 {
                n1479 = Insert Into Array(array=string[] ["1"] ("值"), index=1 ("索引"), new element=w7192) -> (w7190:string[])
                n1480 = call "SQL_Insert.vi"("表名"=w7195, "error in (no error)"=w7196, "值"=w7190, "列名"=string[] ["ST902", "QRCode"], "connection reference"=w7197) -> ("error out"=w7188:errorcluster, "connection reference 2"=w7189:T5)  [unwired: 5 in]
              }
              frame 1, Default {
                n1481 = Decimal String To Number(string=w7207) -> (number=w7206:i32)  [unwired: 2 in, 1 out]
                n1482 = Increment(x=w7206) -> (x+1=w7205:i32)
                n1483 = Number To Decimal String(number=w7205) -> (decimal integer string=w7204:string)  [unwired: 1 in]
                n1484 = Insert Into Array(array=string[] [] ("数组"), index=0 ("索引"), new element=w7204) -> (w7201:string[])
                n1485 = call "SQL_Update.vi"("查询语句"=w7200, "表名"=w7209, "error in (no error)"=w7210, "列名对应的值"=w7201, "列名"=string[] ["ST902"], "connection reference"=w7211) -> ("error out"=w7198:errorcluster, "connection reference 2"=w7199:T5)  [unwired: 4 in]
              }
            }
            n1486 = local read "902二维码"() -> (w7160:string)
            n1487 = Concatenate Strings("Where QRCode='" ("查询语句"), w7160, "'" ("字符串")) -> (w7186:string)
            n1488 = call "SQL_Select.vi"("要读取的列名"=string[] ["Rework_Status"], "表名"="Online", "error in (no error)"=w7143, "查询语句"=w7186, "查询条件"=TRUE, "connection reference"=w7144) -> ("error out"=w7181:errorcluster, "数据"=w7185:string[][], "connection reference out"=w7182:T5)  [unwired: 3 in]
            n1489 = Index Array(array=w7185, index (row)=w7179, index (col)=w7179) -> (element=w7184:string)
            n1490 = Equal?(x=w7184, y="T") -> (x = y?=w7183:bool)
            n1491 = local read "902数据"() -> (w7161:string[])
            n1492 = case shown="真" w7183 {
              tunnel: [w7225 w7235] -> w7171
              tunnel: w7161 -> [w7224 w7238]
              tunnel: [w7219 w7234] -> w7173
              tunnel: w7160 -> [w7218 w7237]
              tunnel: w7186 -> [w7217 w7236]
              tunnel: w7182 -> [w7216 w7249]
              tunnel: w7181 -> [w7215 w7248]
              tunnel: [TRUE w7233] -> w7170
              tunnel: w7142 -> [w7212 w7232]
              frame False {
                n1493 = case shown="\"1\"" w7212 {
                  tunnel: [string[] ["Last_Station", "Last_Result", "ST902_Date", "ST902_Time", "ST902_Result", "ST902_Leakage2", "ST902_Leakage_Upper", "ST902_Leakage_Lower"] string[] ["Last_Station", "Last_Result", "ST902_Date", "ST902_Time", "ST902_Result", "ST902_Leakage3", "ST902_Leakage_Upper", "ST902_Leakage_Lower"] string[] ["Last_Station", "Last_Result", "ST902_Date", "ST902_Time", "ST902_Result", "ST902_Leakage1", "ST902_Leakage_Upper", "ST902_Leakage_Lower"]] -> w7213
                  frame "1" {
                  }
                  frame "2" {
                  }
                  frame "0", Default {
                  }
                }
                n1494 = call "SQL_Update.vi"("查询语句"=w7217, "表名"="Online", "error in (no error)"=w7215, "列名对应的值"=w7224, "列名"=w7213, "connection reference"=w7216) -> ("error out"=w7219:errorcluster)  [unwired: 4 in, 1 out]
                n1495 = Unbundle By Name(w7219) -> ("status"=w7223:bool)
                n1496 = Equal?(x=w7218, y="") -> (x = y?=w7221:bool)
                n1497 = Or(x=w7223, y=w7221) -> (x .or. y?=w7220:bool)
                n1498 = case shown="假" w7220 {
                  tunnel: ["1" ("数据保存请求回复") "2" ("数据保存请求回复")] -> w7225
                  frame False {
                  }
                  frame True {
                  }
                }
              }
              frame True {
                w7244 = 0 ("索引 (行)")
                n1499 = call "SQL_Select.vi"("要读取的列名"=string[] ["[902]"], "表名"="Rework_List", "error in (no error)"=w7248, "查询语句"=w7236, "查询条件"=TRUE, "connection reference"=w7249) -> ("error out"=w7239:errorcluster, "数据"=w7245:string[][], "connection reference out"=w7240:T5)  [unwired: 3 in]
                n1500 = Index Array(array=w7245, index (row)=w7244, index (col)=w7244) -> (element=w7243:string)
                n1501 = Equal?(x=w7243, y="T") -> (x = y?=w7241:bool)
                n1502 = case shown="真" w7241 {
                  tunnel: w7240 -> [w7259 w7283]
                  tunnel: w7239 -> [w7260 w7282]
                  tunnel: w7238 -> [w7258 w7289]
                  tunnel: w7237 -> [w7255 w7284]
                  tunnel: w7236 -> [w7257 w7274]
                  tunnel: [w7254 w7276] -> w7235
                  tunnel: [w7256 w7275] -> w7234
                  tunnel: [TRUE TRUE] -> w7233
                  tunnel: w7232 -> [w7251 w7272]
                  frame False {
                    n1503 = case shown="\"0\", 默认" w7251 {
                      tunnel: [string[] ["Last_Station", "Last_Result", "ST902_Date", "ST902_Time", "ST902_Result", "ST902_Leakage2", "ST902_Leakage_Upper", "ST902_Leakage_Lower"] string[] ["Last_Station", "Last_Result", "ST902_Date", "ST902_Time", "ST902_Result", "ST902_Leakage3", "ST902_Leakage_Upper", "ST902_Leakage_Lower"] string[] ["Last_Station", "Last_Result", "ST902_Date", "ST902_Time", "ST902_Result", "ST902_Leakage1", "ST902_Leakage_Upper", "ST902_Leakage_Lower"]] -> w7252
                      frame "1" {
                      }
                      frame "2" {
                      }
                      frame "0", Default {
                      }
                    }
                    n1504 = call "SQL_Update.vi"("查询语句"=w7257, "表名"="Online", "error in (no error)"=w7260, "列名对应的值"=w7258, "列名"=w7252, "connection reference"=w7259) -> ("error out"=w7256:errorcluster)  [unwired: 4 in, 1 out]
                    n1505 = Unbundle By Name(w7256) -> ("status"=w7264:bool)
                    n1506 = Equal?(x=w7255, y="") -> (x = y?=w7262:bool)
                    n1507 = Or(x=w7264, y=w7262) -> (x .or. y?=w7261:bool)
                    n1508 = case shown="假" w7261 {
                      tunnel: ["1" ("数据保存请求回复") "2" ("数据保存请求回复")] -> w7254
                      frame False {
                      }
                      frame True {
                      }
                    }
                  }
                  frame True {
                    n1509 = Delete From Array(array=w7289, length=2 ("长度"), index=0 ("索引")) -> (deleted portion=w7277:string[], array with subset deleted=w7286:string[])
                    n1510 = call "SQL_Update.vi"("查询语句"=w7274, "表名"="Online", "error in (no error)"=w7282, "列名对应的值"=w7277, "列名"=string[] ["Last_Station", "Last_Result"], "connection reference"=w7283) -> ("error out"=w7281:errorcluster, "connection reference 2"=w7280:T5)  [unwired: 4 in]
                    n1511 = case shown="\"0\", 默认" w7272 {
                      tunnel: [string[] ["ST902_Date", "ST902_Time", "ST902_Result", "ST902_Leakage2", "ST902_Leakage_Upper", "ST902_Leakage_Lower"] string[] ["ST902_Date", "ST902_Time", "ST902_Result", "ST902_Leakage3", "ST902_Leakage_Upper", "ST902_Leakage_Lower"] string[] ["ST902_Date", "ST902_Time", "ST902_Result", "ST902_Leakage1", "ST902_Leakage_Upper", "ST902_Leakage_Lower"]] -> w7271
                      frame "1" {
                      }
                      frame "2" {
                      }
                      frame "0", Default {
                      }
                    }
                    n1512 = call "SQL_Update.vi"("查询语句"=w7274, "表名"="Rework", "error in (no error)"=w7281, "列名对应的值"=w7286, "列名"=w7271, "connection reference"=w7280) -> ("error out"=w7275:errorcluster)  [unwired: 4 in, 1 out]
                    n1513 = Unbundle By Name(w7275) -> ("status"=w7292:bool)
                    n1514 = Equal?(x="", y=w7284) -> (x = y?=w7291:bool)
                    n1515 = Or(x=w7292, y=w7291) -> (x .or. y?=w7290:bool)
                    n1516 = case shown="真" w7290 {
                      tunnel: ["1" ("数据保存请求回复") "2" ("数据保存请求回复")] -> w7276
                      frame False {
                      }
                      frame True {
                      }
                    }
                  }
                }
              }
            }
            "数据保存请求回复902" <- w7171
            n1517 = Delete From Array(array=w7161, length=2 ("长度"), index=0 ("索引")) -> (array with subset deleted=w7168:string[])  [unwired: 1 out]
            n1518 = local write "902数据回复输入"(w7170) -> ()
            n1519 = Insert Into Array(array=w7168, index=2 ("索引"), new element=w7160) -> (w7167:string[])
            n1520 = Insert Into Array(array=string[][] [] ("数组"), index (row)=0 ("索引 (行)"), new element=w7167) -> (w7169:string[][])  [unwired: 1 in]
            n1521 = Transpose 2D Array(2D array=w7169) -> (transposed array=w7159:string[][])
            n1522 = property on="ST902_DATA" class="MCListbox (严格)"("ItemNames"=w7159) -> ()  [unwired: 2 in, 2 out]
            "ST902数据读取（事件）" <- FALSE ("ST902数据读取（事件）")
          }
          event "ST100扫码请求（事件）": Value Change {
            n1523 = event-data() -> ()  [unwired: 1 in, 2 out]
            n1524 = local read "100二维码"() -> (w7299:string)
            n1525 = Concatenate Strings("Where QRCode='" ("查询语句"), w7299, "'" ("字符串")) -> (w7302:string)
            n1526 = call "SQL_Select.vi"("表名"="Online", "error in (no error)"=w7309, "查询语句"=w7302, "查询条件"=TRUE, "connection reference"=w7310) -> ("error out"=w7303:errorcluster, "数据"=w7300:string[][], "connection reference out"=w7304:T5)  [unwired: 4 in]
            n1527 = Matrix Size(0:w7300) -> (1:w7307:i32)  [unwired: 1 out]
            n1528 = Equal To 0?(x=w7307) -> (x = 0?=w7306:bool)
            n1529 = case shown="假" w7306 {
              tunnel: w7304 -> [w7316 w7364]
              tunnel: w7303 -> [w7320 w7363]
              tunnel: w7302 -> [_ w7365]
              tunnel: [w7318 w7358] -> w7301
              tunnel: w7300 -> [w7317 _]
              tunnel: w7299 -> [w7315 _]
              frame False {
                n1530 = case shown="无错误" w7320 {
                  tunnel: [TRUE TRUE] -> w7319
                  tunnel: [w7322 errorcluster {"status"=TRUE, "code"=0, "source"=""} ("error out")] -> w7318
                  tunnel: w7317 -> [w7336 _]
                  tunnel: w7316 -> [w7325 _]
                  tunnel: w7315 -> [w7323 _]
                  frame No Error {
                    n1531 = Index Array(array=w7336, index (row)=0 ("索引 (行)")) -> (element=w7324:string[])  [unwired: 1 in]
                    n1532 = Index Array(array=w7324, index #1=3 ("索引")) -> (element #1=w7333:string, element #2=w7331:string)  [unwired: 1 in]
                    n1533 = local write "扫码请求回复100"("1" ("扫码请求回复100")) -> ()
                    n1534 = local write "上一站结果 (100)"(w7331) -> ()
                    n1535 = local write "上一站号 (100)"(w7333) -> ()
                    n1536 = Equal?(x="902", y=w7333) -> (x = y?=w7328:bool)
                    n1537 = Equal?(x="OK", y=w7331) -> (x = y?=w7329:bool)
                    n1538 = And(x=w7329, y=w7328) -> (x .and. y?=w7327:bool)
                    n1539 = case shown="真" w7327 {
                      tunnel: w7325 -> [_ w7353]
                      tunnel: w7324 -> [_ w7352]
                      tunnel: w7323 -> [_ w7339]
                      tunnel: [errorcluster {"status"=FALSE, "code"=0, "source"=""} ("error out") w7338] -> w7322
                      frame False {
                      }
                      frame True {
                        n1540 = Delete From Array(array=w7352, length=1 ("长度"), index=0 ("索引")) -> (array with subset deleted=w7349:string[])  [unwired: 1 out]
                        n1541 = Format Date/Time String(time format string (%c)="%Y-%m-%d_%H:%M" ("时间格式字符串(%c)")) -> (date/time string=w7346:string)  [unwired: 2 in]
                        n1542 = Replace Array Subset(array=w7349, new element=w7346, index=8 ("索引")) -> (w7345:string[])
                        n1543 = call "SQL_Insert.vi"("表名"="Offline", "值"=w7345, "connection reference"=w7353) -> ("error out"=w7343:errorcluster, "connection reference 2"=w7342:T5)  [unwired: 7 in]
                        n1544 = call "SQL_Delete.vi"("表名"="Online", "error in (no error)"=w7343, "值"=w7339, "列名"="QRCode", "connection reference"=w7342) -> ("error out"=w7338:errorcluster)  [unwired: 5 in, 1 out]
                      }
                    }
                  }
                  frame Error {
                    w7357 = "" ("上一站结果 (100)")
                    n1545 = local write "上一站结果 (100)"(w7357) -> ()
                    n1546 = local write "上一站号 (100)"(w7357) -> ()
                    n1547 = local write "扫码请求回复100"("2" ("扫码请求回复100")) -> ()
                  }
                }
                n1548 = local write "100扫码回复输入"(w7319) -> ()
              }
              frame True {
                n1549 = call "SQL_Select.vi"("要读取的列名"=string[] ["Last_Station", "Last_Result"], "表名"="Offline", "error in (no error)"=w7363, "查询语句"=w7365, "查询条件"=TRUE, "connection reference"=w7364) -> ("error out"=w7358:errorcluster, "数据"=w7359:string[][])  [unwired: 3 in, 1 out]
                n1550 = case shown="无错误" w7358 {
                  tunnel: w7359 -> [w7375 _]
                  tunnel: ["1" ("右扫码请求回复") "2" ("右扫码请求回复")] -> w7360
                  tunnel: [TRUE TRUE] -> w7361
                  frame No Error {
                    n1551 = Index Array(array=w7375, index (row)=0 ("索引 (行)")) -> (element=w7372:string[])  [unwired: 1 in]
                    n1552 = Index Array(array=w7372, index #1=0 ("索引 (行)")) -> (element #1=→"上一站号 (100)":string, element #2=→"上一站结果 (100)":string)  [unwired: 1 in]
                  }
                  frame Error {
                  }
                }
                "扫码请求回复100" <- w7360
                n1553 = local write "100扫码回复输入"(w7361) -> ()
              }
            }
            "ST100扫码请求（事件）" <- FALSE ("ST100扫码请求（事件）")
          }
          event "查询": Value Change {
            n1554 = event-data() -> ()  [unwired: 1 in, 2 out]
            n1555 = flat-sequence {
              tunnel: w7381 -> [w7411]
              tunnel: w7380 -> [w7410]
              tunnel: [w7402] -> w7379
              frame #0 {
                w7382 = cluster{u32, u32}[] [{1985280, 1985280}, {6618880, 6618880}, {1985280, 1985280}, {6618880, 6618880}] ("颜色[4]")
